vi "update DVR pool from nested actors.vi"(9 "Actor number":u32, 10 "Base Actor Queues":T1, 11 "Template in":refnum<class "Template.lvclass">) -> (3 "Template out":refnum<class "Template.lvclass">)   [LabVIEW 2020, in "Template.lvlib" / "Template.lvclass"]
uses:
  Template.lvclass
  typedefs/base actor queues.ctl
  Template.lvclass/Template.ctl
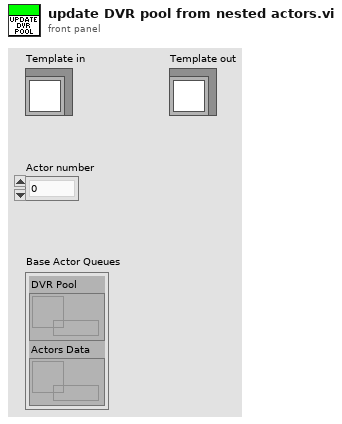
[diagram p1: front panel]
types:
  T1 = typedef "Template.lvlib/Template.lvclass/base actor queues.ctl" = cluster{"DVR Pool":refnum<queue>, "Actors Data":refnum<queue>}
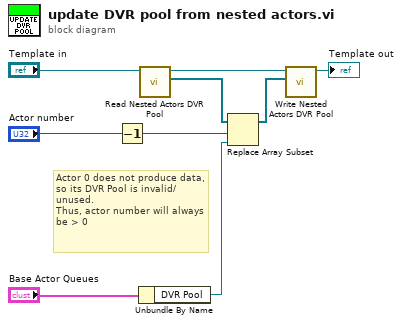
[diagram p0: block diagram]
diagram:
  # "Actor 0 does not produce data, so its DVR Pool is invalid/unused.\nThus, actor number will always be > 0"
  n1 = Decrement(x="Actor number") -> (x-1=w3:u32)
  n2 = Unbundle By Name("Base Actor Queues") -> ("DVR Pool"=w2:refnum<queue>)
  n3 = call "Read Nested Actors DVR Pool.vi"("Template in"="Template in") -> ("Nested Actors DVR Pool"=w4:refnum<queue>[], "Template out"=w5:refnum<class "Template.lvclass">)  [unwired: 9 in]
  n4 = Replace Array Subset(array=w4, new element=w2, index=w3) -> (w1:refnum<queue>[])
  n5 = call "Write Nested Actors DVR Pool.vi"("Nested Actors DVR Pool"=w1, "Template in"=w5) -> ("Template out"=→"Template out":refnum<class "Template.lvclass">)  [unwired: 9 in]
